vi "Create.vi"(5 "Param Class":string, 7 "Param Event":refnum<user-event>, 8 "error in (no error)":errorcluster, 9 "Result Reg":refnum<event-registration>, 10 "Result Event":refnum<user-event>, 11 "Result Class":string) -> (0 "error out":errorcluster, 3 "Future out":refnum<class "Future.lvclass">)   [LabVIEW 2020, in "Promises.lvlib" / "Future.lvclass"]
uses:
  Future.lvclass
  Result.ctl
  Result State.ctl
  Parameter Data.ctl
  Future.lvclass/Future.ctl
  Promises.lvlib
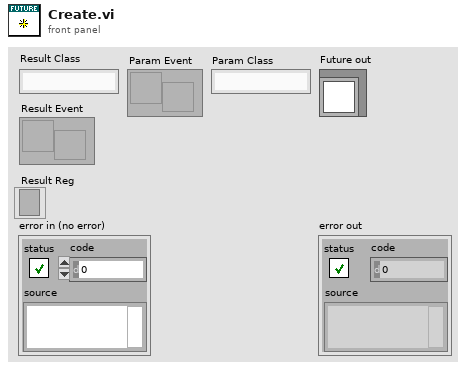
[diagram p1: front panel]
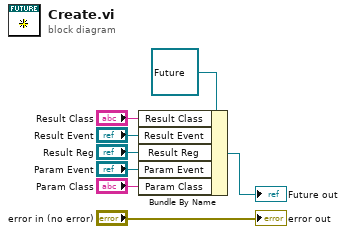
[diagram p0: block diagram]
diagram:
  n1 = Bundle By Name(cluster=refnum<class "Future.lvclass"> refnum ("Future in"), "Result Class"="Result Class", "Result Event"="Result Event", "Result Reg"="Result Reg", "Param Event"="Param Event", "Param Class"="Param Class") -> (→"Future out":refnum<class "Future.lvclass">)
  "error out" <- "error in (no error)"
